vi "mqttStartDaemon.vi"(8 "error in (no error)":errorcluster, 11 "mqtt in":refnum<class "mqtt.lvclass">) -> (0 "error out":errorcluster, 3 "mqtt out":refnum<class "mqtt.lvclass">)   [LabVIEW 2018, in "labview-mqtt.lvlib" / "mqtt.lvclass"]
uses:
  mqtt.lvclass
  mqttTCPIPserver.vi
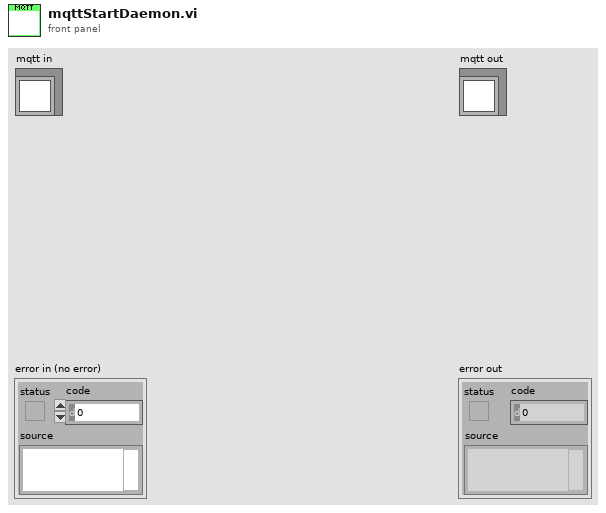
[diagram p1: front panel]
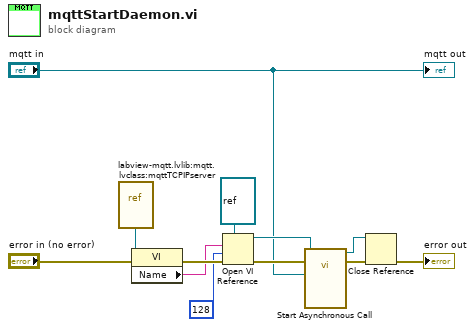
[diagram p0: block diagram]
diagram:
  n1 = vi-ref "labview-mqtt.lvlib:mqtt.lvclass:mqttTCPIPserver.vi"() -> (w10:refnum<vi>)
  n2 = property class="VI"(reference=w10, error in="error in (no error)") -> (error out=w11:errorcluster, "Name"=w8:string)  [unwired: 1 out]
  n3 = Open VI Reference(type specifier VI Refnum (for type only)=refnum<vi> refnum, vi path=w8, options=128, error in (no error)=w11) -> (vi reference=w5:refnum<vi>, error out=w9:errorcluster)  [unwired: 2 in]
  n4 = call-by-ref "Start Asynchronous Call"(reference=w5, error in=w9, "mqtt.lvclass"="mqtt in") -> (reference out=w3:refnum<vi>, error out=w6:errorcluster)  [unwired: 13 in, 2 out]
  n5 = Close Reference(reference=w3, error in (no error)=w6) -> (error out=→"error out":errorcluster)
  "mqtt out" <- "mqtt in"
